vi "Get Type.vi"(8 "error in (no error)":errorcluster, 11 "Node in":refnum<class "Node.lvclass">) -> (0 "error out":errorcluster, 2 "Node Type":T1, 3 "Node out":refnum<class "Node.lvclass">)   [LabVIEW 2020, in "PicoG-ParserLexer.lvlib" / "Node.lvclass"]
uses:
  Node.lvclass
  AST Node Type.ctl
  PicoG-ParserLexer.lvlib
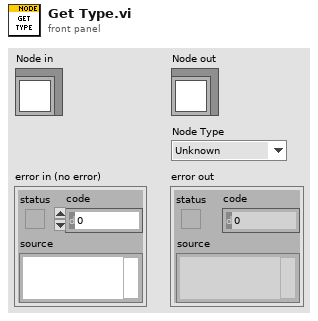
[diagram p1: front panel]
types:
  T1 = typedef "PicoG-ParserLexer.lvlib/AST Node Type.ctl" = enum16{"Unknown", "Keyword", "Array", "Cluster", "Numeric", "Boolean", "String", "Identifier"}
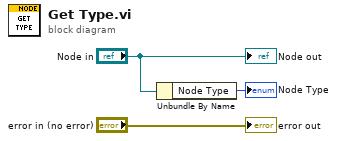
[diagram p0: block diagram]
diagram:
  n1 = Unbundle By Name("Node in") -> ("Node Type"=→"Node Type":T1)
  "error out" <- "error in (no error)"
  "Node out" <- "Node in"
